vi "Post_X_Field_Every_T.vi"() -> ()   [LabVIEW 2013]
panel:
  in  "stop":bool
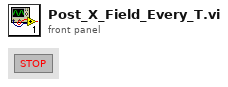
[diagram p1: front panel]
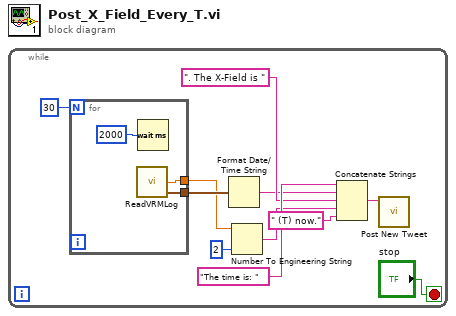
[diagram p0: block diagram]
diagram:
  n1 = while {
    stop <- "stop" stop-if-true
    n2 = for {
      N: 30 -> [_]
      tunnel: [w14] -> w9
      tunnel: [w13] -> w8
      n3 = call "ReadVRMLog.vi"() -> ("time stamp"=w14:timestamp, "X Field"=w13:dbl)  [unwired: 4 in]
      n4 = Wait (ms)(milliseconds to wait=u32 2000) -> ()  [unwired: 1 out]
    }
    n5 = Format Date/Time String(seconds (now)=w9) -> (date/time string=w4:string)  [unwired: 2 in]
    n6 = Number To Engineering String(2:i16 2 ("precision (6)"), 4:w8) -> (0:w2:string)  [unwired: 2 in]
    n7 = Concatenate Strings("The time is: " ("string"), w4, ". The X-Field is " ("string"), w2, " (T) now." ("string")) -> (w7:string)
    n8 = call "Post New Tweet.vi"("Message Main Body"=w7) -> ()  [unwired: 11 in]
  }
